vi "ex01_e.vi"() -> ()   [LabVIEW 2011]
panel:
  in  "stop":bool
  out "String 2":string
  in  "String":string
  out "Boolean 3":bool
  in  "OK Button":bool
  in  "Boolean 2":bool
  out "Numeric Indicator":i64
  in  "Numeric Control":dbl
  out "Boolean":bool
  out "Gauge":dbl(knob) scale=0.1..100.0
  in  "Knob":dbl(knob) scale=0.0..100.0
  out "Numeric 2":dbl
  in  "Numeric":dbl
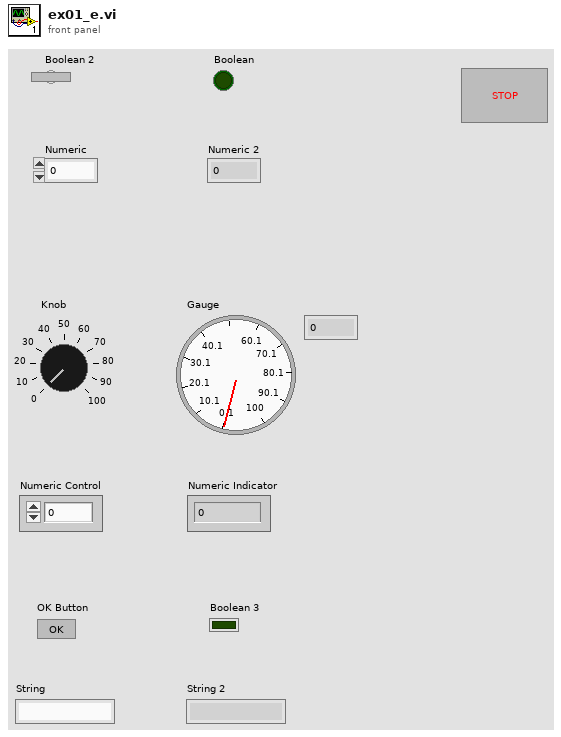
[diagram p1: front panel]
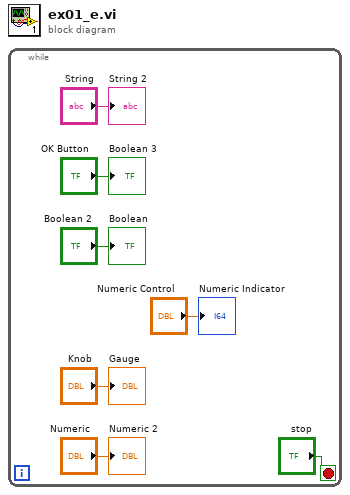
[diagram p0: block diagram]
diagram:
  n1 = while {
    stop <- "stop" stop-if-true
    "Numeric 2" <- "Numeric"
    "Gauge" <- "Knob"
    "Boolean" <- "Boolean 2"
    "Numeric Indicator" <- "Numeric Control"
    "Boolean 3" <- "OK Button"
    "String 2" <- "String"
  }
